vi "runtime io test.vi"() -> ()   [LabVIEW 2013, in "sample module tests.lvlib"]
uses:
  sample module tests.lvlib
  module/execution/sample module runtime.lvclass
  <vilib>/NI/Tag Bus/tag/tag descriptor.lvclass/tag descriptor.ctl
  <vilib>/NI/Tag Bus/table/data polymorphs/write one/write Double.vi
  <vilib>/NI/Tag Bus/table/data polymorphs/read one/read Double.vi
  <vilib>/NI/Tag Bus/tag/read tag name.vi
  <vilib>/NI/Tag Bus/tag/read data type.vi
  <vilib>/NI/Tag Bus/dictionary/data dictionary.lvclass
  channel/TBM channel.lvclass
  <vilib>/NI/Tag Bus/table/data table.lvlib
panel:
  out "inputs changed?":bool
  out "no error":errorcluster
  # "This is expected to remain false until you write code for input"
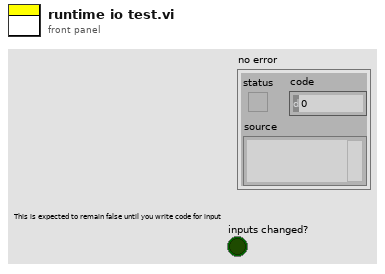
[diagram p1: front panel]
types:
  T1 = typedef "TBM channel.lvclass/data tables.ctl" = cluster{"input data":T2, "processing parameter":T2, "processing result":T2, "output data":T2}
  T2 = typedef "tag bus.lvlib/dictionary table pair.ctl" = cluster{"data dictionary":refnum<class "data dictionary.lvclass">, "data table":T3}
  T3 = typedef "tag bus.lvlib/data table.lvlib/data table.ctl" = cluster{"Double":dbl[], "Single":sgl[], "I64":i64[], "I32":i32[], "I16":i16[], "I8":i8[], "U64":u64[], "U32":u32[], "U16":u16[], "U8":u8[], "Boolean":bool[], "String":string[], "Array of Double":cluster{"DBL Array":dbl[]}[], "Array of Single":cluster{"SGL Array":sgl[]}[], "Array of I64":cluster{"I64 Array":i64[]}[], "Array of I32":cluster{"I32 Array":i32[]}[], "Array of I16":cluster{"I16 Array":i16[]}[], "Array of I8":cluster{"I8 Array":i8[]}[], "Array of U64":cluster{"U64 Array":u64[]}[], "Array of U32":cluster{"U32 Array":u32[]}[], "Array of U16":cluster{"U16 Array":u16[]}[], "Array of U8":cluster{"U8 Array":u8[]}[], "Array of Boolean":cluster{"Boolean Array":bool[]}[], "Array of String":cluster{"String Array":string[]}[]}
  T4 = typedef "tag bus.lvlib/tag descriptor.lvclass/Data Type.ctl" = enum16{"Double", "Single", "I64", "I32", "I16", "I8", "U64", "U32", "U16", "U8", "Boolean", "String", "Array of Double", "Array of Single", "Array of I64", "Array of I32", "Array of I16", "Array of I8", "Array of U64", "Array of U32", "Array of U16", "Array of U8", "Array of Boolean", "Array of String"}
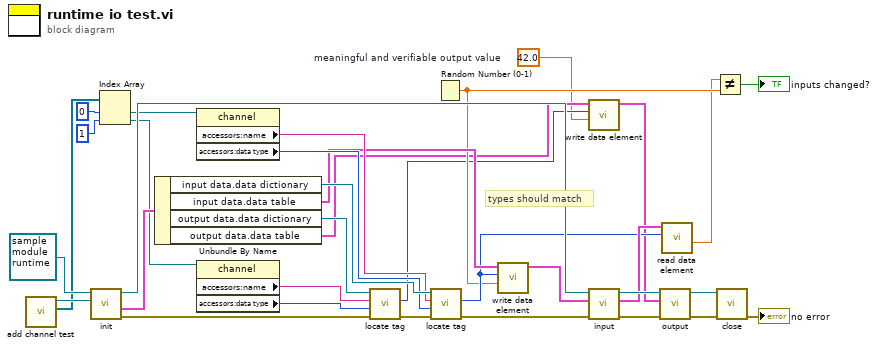
[diagram p0: block diagram]
diagram:
  w3 = 42.0  # meaningful and verifiable output value
  # "types should match"
  n1 = call "add channel test.vi"() -> ("channels"=w1:refnum<class "TBM channel.lvclass">[], "sample module configuration out"=w2:refnum<class "sample module configuration.lvclass">)  [unwired: 8 in, 2 out]
  n2 = call-dynamic "init.vi"("module configuration"=w2, "module in"=refnum<class "sample module runtime.lvclass"> refnum ("sample module")) -> ("error out"=w8:errorcluster, "data allocations"=w25:T1, "module out"=w26:refnum<class "sample module runtime.lvclass">)  [unwired: 6 in, 1 out]
  n3 = Index Array(array=w1, index #1=0 ("index (row)"), index #2=1 ("index (row)")) -> (element #1=w23:refnum<class "TBM channel.lvclass">, element #2=w12:refnum<class "TBM channel.lvclass">)
  n4 = Unbundle By Name(w25) -> ("input data.data dictionary"=w24:refnum<class "data dictionary.lvclass">, "input data.data table"=w20:T3, "output data.data dictionary"=w11:refnum<class "data dictionary.lvclass">, "output data.data table"=w6:T3)
  n5 = property class="channel"(reference=w23) -> ("accessors:name"=w21:string, "accessors:data type"=w22:T4)  [unwired: 1 in, 2 out]
  n6 = property class="channel"(reference=w12) -> ("accessors:name"=w10:string, "accessors:data type"=w9:T4)  [unwired: 1 in, 2 out]
  n7 = call <vilib>:"locate tag.vi"("error in"=w8, "data type"=w9, "name"=w10, "data dictionary in"=w11) -> ("error out"=w7:errorcluster, "index"=w4:i32)  [unwired: 5 in, 1 out]
  n8 = call <vilib>:"locate tag.vi"("error in"=w7, "data type"=w22, "name"=w21, "data dictionary in"=w24) -> ("error out"=w18:errorcluster, "index"=w16:i32)  [unwired: 5 in, 1 out]
  n9 = Random Number (0-1)() -> (number: 0 to 1=w15:dbl)
  n10 = call-poly <vilib>:"write data element.vi"("value"=w15, "index"=w16, "data table in"=w20) -> ("data table out"=w19:T3)  [unwired: 8 in]
  n11 = call-poly <vilib>:"write data element.vi"("value"=w3, "index"=w4, "data table in"=w6) -> ("data table out"=w5:T3)  [unwired: 8 in]
  n12 = call-dynamic "input.vi"("error in"=w18, "input allocation"=w19, "module in"=w26) -> ("error out"=w27:errorcluster, "input data"=w17:T3, "module out"=w28:refnum<class "sample module runtime.lvclass">)  [unwired: 6 in]
  n13 = call-dynamic "output.vi"("error in"=w27, "output data"=w5, "module in"=w28) -> ("error out"=w29:errorcluster, "module out"=w30:refnum<class "sample module runtime.lvclass">)  [unwired: 6 in, 1 out]
  n14 = call-poly <vilib>:"read data element.vi"("index"=w16, "data table in"=w17) -> ("value"=w14:dbl)  [unwired: 8 in, 1 out]
  n15 = Not Equal?(x=w14, y=w15) -> (x != y?=→"inputs changed?":bool)
  n16 = call-dynamic "close.vi"("error in"=w29, "module in"=w30) -> ("error out"=→"no error":errorcluster)  [unwired: 9 in]
